vi "_script_vi_paths.vi"(8 "error in (no error)":errorcluster, 11 "Directory":path) -> (0 "error out":errorcluster, 3 "VI Paths":path[](array[path]))   [LabVIEW 2019, in "Script.lvlib"]
doc: "Returns the array of plugin VI paths in the _Scripts directory.\n\nCreated by: Ryan Pacini"
uses:
  Script.lvlib
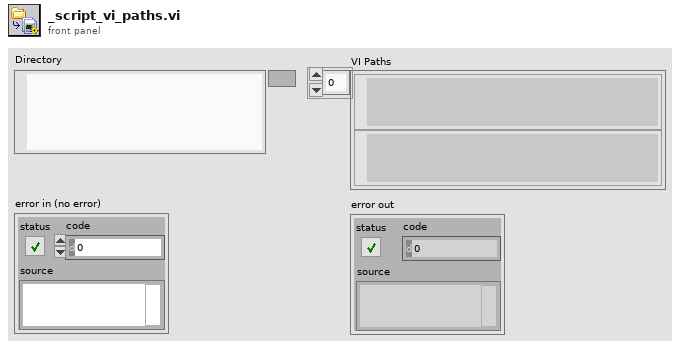
[diagram p1: front panel]
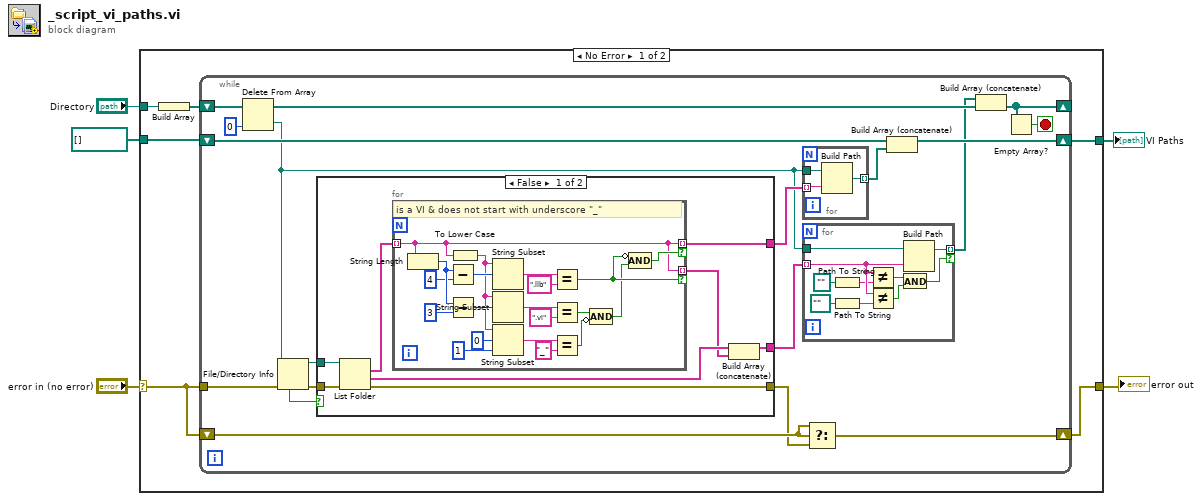
[diagram p0: block diagram]
diagram:
  n1 = case shown="No Error" "error in (no error)" {
    selector: "error in (no error)" -> [w7 w74]
    tunnel: "Directory" -> [w11 _]
    tunnel: [w8 w73] -> w5
    tunnel: [w9 w74] -> w3
    tunnel: path[] [] ("Array Constant") -> [w6 w73]
    frame No Error {
      n2 = Build Array(w11) -> (w10:path[])
      n3 = while {
        shift-left: w6 -> [w28]
        shift-right: [w30] -> w8
        shift-left: w10 -> [w29]
        shift-right: [w27] -> _
        shift-right: [w24] -> w9
        shift-left: w7 -> [w23]
        tunnel: w7 -> [w13]
        stop <- w26 stop-if-true
        n4 = Delete From Array(array=w29, index=0) -> (deleted portion=w12:path, array with subset deleted=w22:path[])  [unwired: 1 in]
        n5 = File/Directory Info(path=w12, error in=w13) -> (path out=w19:path, error out=w20:errorcluster, shortcut=w18:bool)  [unwired: 4 out]
        n6 = case shown="False" w18 {
          tunnel: [w35 _] -> w16
          tunnel: [w34 w59] -> w17
          tunnel: [w32 _] -> w21
          tunnel: w20 -> [w38 w59]
          tunnel: w19 -> [w37 _]
          frame False {
            n7 = List Folder(path=w37, error in=w38) -> (filenames=w36:string[], folder names=w33:string[], error out=w34:errorcluster)  [unwired: 1 in, 2 out]
            n8 = for {
              tunnel: w36 -> [w51] mode=indexing
              tunnel: [w51] -> w35 mode=indexing if=w55
              tunnel: [w51] -> w31 mode=indexing if=w56
              # "is a VI & does not start with underscore \"_\""
              n9 = String Length(string=w51) -> (length=w52:i32)
              n10 = Subtract(x=w52, y=4) -> (x-y=w58:i32)
              n11 = Subtract(x=w52, y=3) -> (x-y=w53:i32)
              n12 = To Lower Case(string=w51) -> (all lower case string=w48:string)
              n13 = String Subset(string=w48, offset (0)=w58) -> (substring=w49:string)  [unwired: 1 in]
              n14 = String Subset(string=w48, offset (0)=w53) -> (substring=w50:string)  [unwired: 1 out]
              n15 = String Subset(string=w48, offset (0)=0, length (rest)=1 ("length (rest)")) -> (substring=w46:string)
              n16 = Equal?(x=w49, y=".llb") -> (x = y?=w56:bool)
              n17 = Equal?(x=w50, y=".vi") -> (x = y?=w45:bool)
              n18 = Equal?(x=w46, y="_") -> (x = y?=w43:bool)
              n19 = Compound Arithmetic op=AND(w45, invert w43) -> (w39:bool)
              n20 = Compound Arithmetic op=AND(invert w56, w39) -> (w55:bool)
            }
            n21 = Build Array (concatenate)(w33, w31) -> (w32:string[])
          }
          frame True {
          }
        }
        n22 = for {
          tunnel: w16 -> [w71] mode=indexing
          tunnel: w12 -> [w72]
          tunnel: [w70] -> w14 mode=indexing
          n23 = Build Path(base path=w72, name or relative path=w71) -> (appended path=w70:path)
        }
        n24 = for {
          tunnel: w12 -> [w69]
          tunnel: [w68] -> w15 mode=indexing if=w67
          tunnel: w21 -> [w66] mode=indexing
          n25 = Path To String(path=path "") -> (string=w62:string)
          n26 = Path To String(path=path "..") -> (string=w60:string)
          n27 = Not Equal?(x=w66, y=w62) -> (x != y?=w64:bool)
          n28 = Not Equal?(x=w66, y=w60) -> (x != y?=w65:bool)
          n29 = And(x=w64, y=w65) -> (x .and. y?=w67:bool)
          n30 = Build Path(base path=w69, name or relative path=w66) -> (appended path=w68:path)
        }
        n31 = Select(t=w23, s=w23, f=w17) -> (s? t:f=w24:errorcluster)
        n32 = Build Array (concatenate)(w28, w14) -> (w30:path[])
        n33 = Build Array (concatenate)(w15, w22) -> (w27:path[])
        n34 = Empty Array?(array=w27) -> (empty?=w26:bool)
      }
    }
    frame Error {
    }
  }
  "VI Paths" <- w5
  "error out" <- w3
